vi "LN_GetNextNodeRef.vi"(3 "InputListNode":refnum<class "ListNode.lvclass">) -> (0 "OutputNextNodeRef":refnum<data-value>, 1 "OutputListNode":refnum<class "ListNode.lvclass">)   [LabVIEW 2014, in "ListNode.lvclass"]
uses:
  ListNode.lvclass
  ListNodeVirtual.lvclass
  ListNode.lvclass/ListNode.ctl
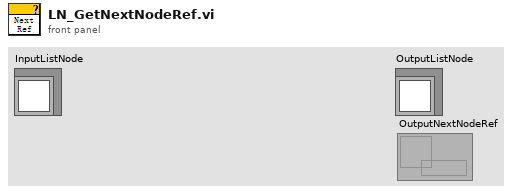
[diagram p1: front panel]
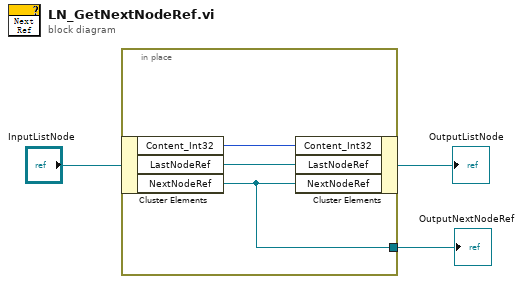
[diagram p0: block diagram]
diagram:
  n1 = in-place {
    in-place-border: [w4] -> w1
    n2 = in-place-cluster #1("InputListNode") -> ("Content_Int32"=w6:i32, "LastNodeRef"=w5:refnum<data-value>, "NextNodeRef"=w4:refnum<data-value>)
    n3 = in-place-cluster #1("Content_Int32"=w6, "LastNodeRef"=w5, "NextNodeRef"=w4) -> (→"OutputListNode":refnum<class "ListNode.lvclass">)
  }
  "OutputNextNodeRef" <- w1
